vi "computeCentroid.vi"(11 "locations":cluster{"X":sgl, "Y":sgl, "Z":sgl}[](array[cluster])) -> (2 "median":cluster{"X":sgl, "Y":sgl, "Z":sgl}, 4 "SDradius":dbl format="%0.2f", 6 "meanRadius":dbl format="%0.2f")   [LabVIEW 2022 SP3]
uses:
  <vilib>/Analysis/baseanly.llb/Real Dot Product.vi
  <vilib>/Analysis/NI_AALBase.lvlib
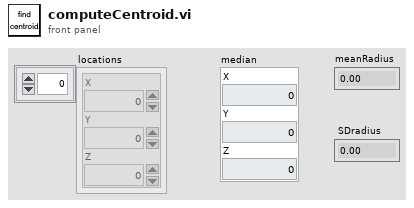
[diagram p1: front panel]
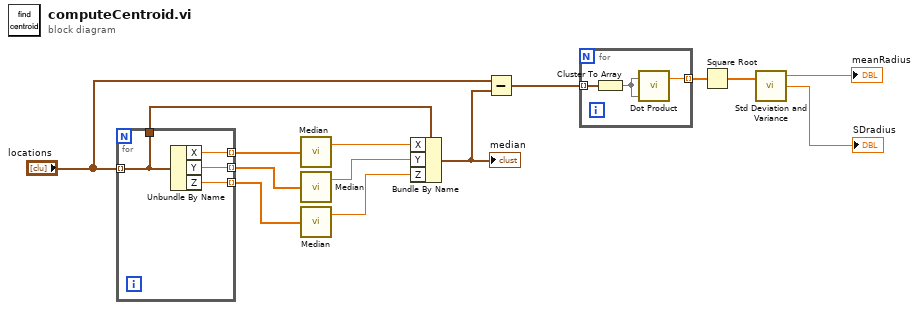
[diagram p0: block diagram]
diagram:
  n1 = for {
    tunnel: "locations" -> [w15] mode=indexing
    tunnel: [w18] -> w14 mode=indexing
    tunnel: [w17] -> w13 mode=indexing
    tunnel: [w16] -> w12 mode=indexing
    tunnel: [w15] -> w8
    n2 = Unbundle By Name(w15) -> ("X"=w18:sgl, "Y"=w17:sgl, "Z"=w16:sgl)
  }
  n3 = call <vilib>:"Median.vi"("X"=w14) -> ("median"=w11:dbl)  [unwired: 1 out]
  n4 = call <vilib>:"Median.vi"("X"=w13) -> ("median"=w10:dbl)  [unwired: 1 out]
  n5 = call <vilib>:"Median.vi"("X"=w12) -> ("median"=w9:dbl)  [unwired: 1 out]
  n6 = Bundle By Name(cluster=w8, "X"=w11, "Y"=w10, "Z"=w9) -> (w7:cluster{"X":sgl, "Y":sgl, "Z":sgl})
  "median" <- w7
  n7 = Subtract(x="locations", y=w7) -> (x-y=w5:cluster{"X":sgl, "Y":sgl, "Z":sgl}[])
  n8 = for {
    tunnel: w5 -> [w21] mode=indexing
    tunnel: [w19] -> w4 mode=indexing
    n9 = Cluster To Array(cluster=w21) -> (array=w20:sgl[])
    n10 = call-poly <vilib>:"Dot Product.vi"("Y Vector"=w20, "X Vector"=w20) -> ("X * Y"=w19:dbl)  [unwired: 1 out]
  }
  n11 = Square Root(x=w4) -> (sqrt(x)=w1:dbl[])
  n12 = call <vilib>:"Std Deviation and Variance.vi"("X"=w1) -> ("mean"=→"meanRadius":dbl, "standard deviation"=→"SDradius":dbl)  [unwired: 1 in, 1 out]
